vi "Engine - PFI - Sensors Host.vi"() -> ()   [LabVIEW 2015, in "ECS-Host.lvlib"]
uses:
  ECS-Host.lvlib
  <vilib>/addons/Software Calibration Management/XControls/TBL1D.xctl
panel:
  in  "_Tab Control":enum32{"Pressures", "Temperatures", "Other"}(tab)
  out "MAP":sgl caption="[]"
  out "MAP_Raw":sgl caption="[]"
  in  "MAP_Sim":sgl caption="[]"
  in  "MAP_SimE":bool
  in  "MAP_FiltInit":bool
  in  "MAP_FiltE":bool
  in  "MAP_FiltBreak":sgl caption="[]"
  in  "MAP_Tbl":cluster{"X":sgl[], "Y":sgl[]}(xcontrol) caption="[]"
  out "FuelP":sgl caption="[]"
  out "FuelP_Raw":sgl caption="[]"
  in  "FuelP_Sim":sgl caption="[]"
  in  "FuelP_SimE":bool
  in  "FuelP_FiltInit":bool
  in  "FuelP_FiltE":bool
  in  "FuelP_FiltBreak":sgl caption="[]"
  in  "FuelP_Tbl":cluster{"X":sgl[], "Y":sgl[]}(xcontrol) caption="[]"
  out "CACOutP":sgl caption="[]"
  out "CACOutP_Raw":sgl caption="[]"
  in  "CACOutP_Sim":sgl caption="[]"
  in  "CACOutP_SimE":bool
  in  "CACOutP_FiltInit":bool
  in  "CACOutP_FiltE":bool
  in  "CACOutP_FiltBreak":sgl caption="[]"
  in  "CACOutP_Tbl":cluster{"X":sgl[], "Y":sgl[]}(xcontrol) caption="[]"
  out "BaroAirP":sgl caption="[]"
  out "BaroAirP_Raw":sgl caption="[]"
  in  "BaroAirP_Sim":sgl caption="[]"
  in  "BaroAirP_SimE":bool
  in  "BaroAirP_FiltInit":bool
  in  "BaroAirP_FiltE":bool
  in  "BaroAirP_FiltBreak":sgl caption="[]"
  in  "BaroAirP_Tbl":cluster{"X":sgl[], "Y":sgl[]}(xcontrol) caption="[]"
  in  "OilP_Tbl":cluster{"X":sgl[], "Y":sgl[]}(xcontrol) caption="[]"
  in  "OilP_FiltBreak":sgl caption="[]"
  in  "OilP_FiltE":bool
  in  "OilP_FiltInit":bool
  in  "OilP_SimE":bool
  in  "OilP_Sim":sgl caption="[]"
  out "OilP_Raw":sgl caption="[]"
  out "OilP":sgl caption="[]"
  in  "IntakeAirT_Tbl":cluster{"X":sgl[], "Y":sgl[]}(xcontrol) caption="[]"
  in  "IntakeAirT_FiltBreak":sgl caption="[]"
  in  "IntakeAirT_FiltE":bool
  in  "IntakeAirT_FiltInit":bool
  in  "IntakeAirT_SimE":bool
  in  "IntakeAirT_Sim":sgl caption="[]"
  out "IntakeAirT_Raw":sgl caption="[]"
  out "IntakeAirT":sgl caption="[]"
  in  "MAT_Tbl":cluster{"X":sgl[], "Y":sgl[]}(xcontrol) caption="[]"
  in  "MAT_FiltBreak":sgl caption="[]"
  in  "MAT_FiltE":bool
  in  "MAT_FiltInit":bool
  in  "MAT_SimE":bool
  in  "MAT_Sim":sgl caption="[]"
  out "MAT_Raw":sgl caption="[]"
  out "MAT":sgl caption="[]"
  in  "FuelT_Tbl":cluster{"X":sgl[], "Y":sgl[]}(xcontrol) caption="[]"
  in  "FuelT_FiltBreak":sgl caption="[]"
  in  "FuelT_FiltE":bool
  in  "FuelT_FiltInit":bool
  in  "FuelT_SimE":bool
  in  "FuelT_Sim":sgl caption="[]"
  out "FuelT_Raw":sgl caption="[]"
  out "FuelT":sgl caption="[]"
  out "ECT":sgl caption="[]"
  out "ECT_Raw":sgl caption="[]"
  in  "ECT_Sim":sgl caption="[]"
  in  "ECT_SimE":bool
  in  "ECT_FiltInit":bool
  in  "ECT_FiltE":bool
  in  "ECT_FiltBreak":sgl caption="[]"
  in  "ECT_Tbl":cluster{"X":sgl[], "Y":sgl[]}(xcontrol) caption="[]"
  out "TDKBattV":sgl caption="[]"
  out "5VPulsBattV":sgl caption="[]"
  out "12VPulsBattV":sgl caption="[]"
  in  "MAF_Tbl":cluster{"X":sgl[], "Y":sgl[]}(xcontrol) caption="[]"
  in  "MAF_FiltBreak":sgl caption="[]"
  in  "MAF_FiltE":bool
  in  "MAF_FiltInit":bool
  in  "MAF_SimE":bool
  in  "MAF_Sim":sgl caption="[]"
  out "MAF_Raw":sgl caption="[]"
  out "MAF":sgl caption="[]"
  out "Pedal":sgl caption="[]"
  out "Pedal_Raw":sgl caption="[]"
  in  "Pedal_Sim":sgl caption="[]"
  in  "Pedal_SimE":bool
  in  "Pedal_FiltInit":bool
  in  "Pedal_FiltE":bool
  in  "Pedal_FiltBreak":sgl caption="[]"
  in  "Pedal_Tbl":cluster{"X":sgl[], "Y":sgl[]}(xcontrol) caption="[]"
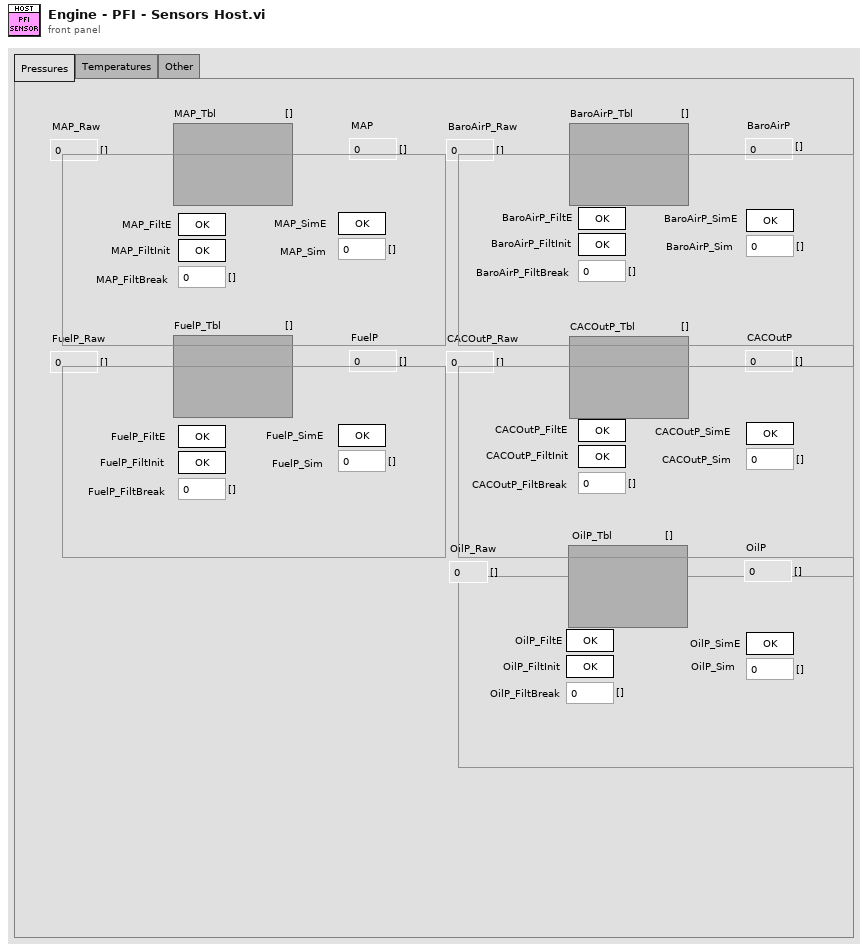
[diagram p1: front panel]
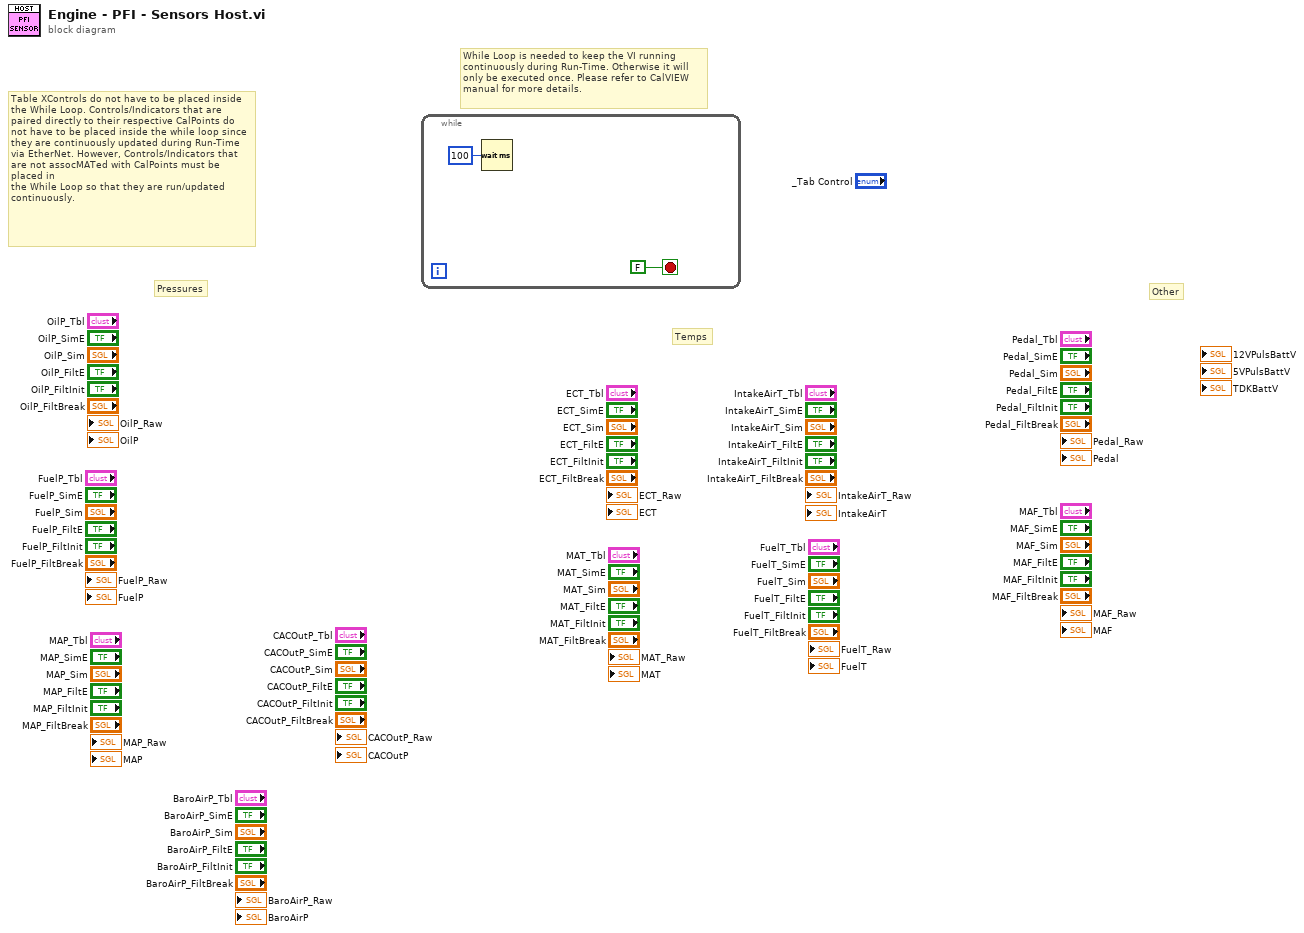
[diagram p0: block diagram]
diagram:
  # "Other"
  # "Temps"
  # "Pressures"
  # "Table XControls do not have to be placed inside the While Loop. Controls/Indicators that are paired directly to their respective CalPoints do not have to be placed inside the while loop since they are continuously updated during Run-Time via EtherNet. However, Controls/Indicators that are not assocMATed with CalPoints must be placed in\nthe While Loop so that they are run/updated continuously."
  # "While Loop is needed to keep the VI running\ncontinuously during Run-Time. Otherwise it will only be executed once. Please refer to CalVIEW manual for more details."
  n1 = while {
    stop <- FALSE stop-if-true
    n2 = Wait (ms)(milliseconds to wait=u32 100) -> ()  [unwired: 1 out]
  }
